vi "UpdateNativePropertyMethod.vi"(1 "VI":refnum<vi>, 2 "TypeDefControl":path=path "C:/classes/ObjectAttributes.ctl", 3 "Property":string, 5 "error IO":errorcluster, 6 "GetMethod":bool) -> (19 "error out":errorcluster)   [LabVIEW 2012, in "ClassWriterNative.lvclass"]
uses:
  <resource>/Framework/Providers/Open_GDS/ClassProviders/Provider_LvNativeClass/ClassWriterNative_class/ClassWriterNative.lvclass
  <vilib>/Utility/miscctls.llb/LVPositionTypeDef.ctl
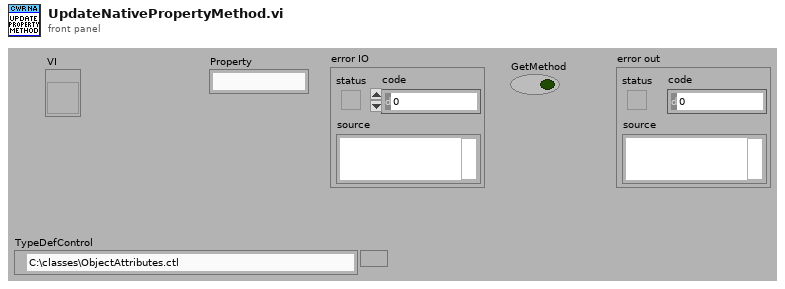
[diagram p1: front panel]
types:
  T1 = typedef "LVPositionTypeDef.ctl" = cluster{"Left":i32, "Top":i32}
  T2 = enum16{"Invalid Wire Rule", "Required", "Recommended", "Optional", "Dynamic Dispatch"}
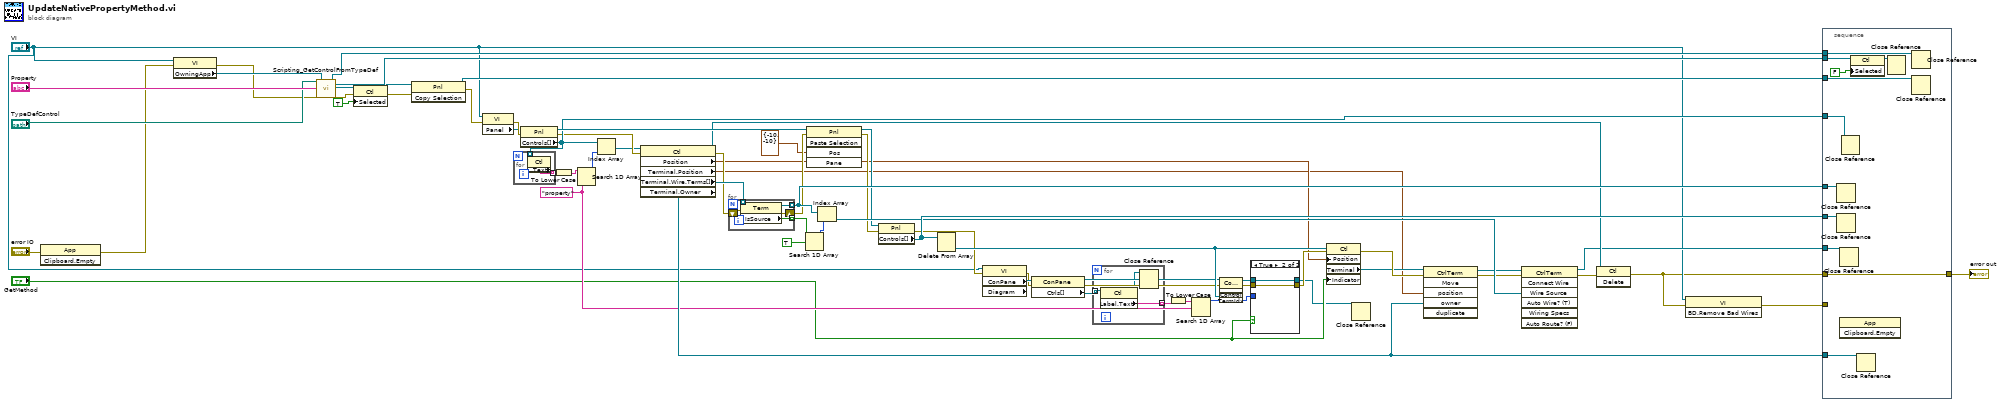
[diagram p0: block diagram]
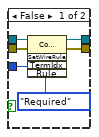
[diagram p2: hidden frame]
diagram:
  w16 = "property" ("element")
  n1 = invoke class="App" method="Clipboard.Empty"(error in="error IO") -> (error out=w5:errorcluster)  [unwired: 2 in, 2 out]
  n2 = property class="VI"(reference="VI", error in=w5) -> (error out=w4:errorcluster, "OwningApp"=w6:refnum<vi>)  [unwired: 1 out]
  n3 = call <resource>:"Scripting_GetControlFromTypeDef.vi"("TypeDefControl"="TypeDefControl", "String"="Property", "error in"=w4, "AppRef"=w6) -> ("vi reference"=w21:refnum<vi>, "Panel"=w20:refnum<vi>, "ControlRef"=w40:refnum<vi>, "error out"=w42:errorcluster)  [unwired: 12 in]
  n4 = property class="Ctl"(reference=w40, error in=w42, "Selected"=TRUE) -> (reference out=w58:refnum<vi>, error out=w41:errorcluster)
  n5 = invoke class="Pnl" method="Copy Selection"(reference=w20, error in=w41) -> (reference out=w57:refnum<vi>, error out=w43:errorcluster)  [unwired: 1 in, 1 out]
  n6 = property class="VI"(reference="VI", error in=w43) -> (error out=w45:errorcluster, "Panel"=w44:refnum<vi>)  [unwired: 1 out]
  n7 = property class="Pnl"(reference=w44, error in=w45) -> (reference out=w63:refnum<vi>, error out=w49:errorcluster, "Controls[]"=w59:refnum<vi>[])
  n8 = for {
    tunnel: w59 -> [w68] mode=indexing
    tunnel: [w67] -> w46 mode=indexing
    n9 = property class="Ctl"(reference=w68) -> ("Label.Text"=w67:string)  [unwired: 1 in, 2 out]
  }
  n10 = To Lower Case(string=w46) -> (all lower case string=w62:string[])
  n11 = Search 1D Array(1D array=w62, element=w16) -> (index of element=w47:i32)  [unwired: 1 in]
  n12 = Index Array(array=w59, index=w47) -> (element=w48:refnum<vi>)
  n13 = property class="Ctl"(reference=w48, error in=w49) -> (reference out=w34:refnum<vi>, error out=w37:errorcluster, "Position"=w29:T1, "Terminal.Position"=w24:T1, "Terminal.Wire.Terms[]"=w50:refnum<vi>[], "Terminal.Owner"=w22:refnum<vi>)
  n14 = for {
    tunnel: w50 -> [w73] mode=indexing
    tunnel: [w72] -> w51 mode=indexing
    tunnel: [w71] -> w60 mode=indexing
    shift-right: [w69] -> w36
    shift-left: w37 -> [w70]
    n15 = property class="Term"(reference=w73, error in=w70) -> (reference out=w71:refnum<vi>, error out=w69:errorcluster, "IsSource"=w72:bool)
  }
  n16 = Search 1D Array(1D array=w51, element=TRUE) -> (index of element=w53:i32)  [unwired: 1 in]
  n17 = invoke class="Pnl" method="Paste Selection"(reference=w63, error in=w36, "Pos"=T1 {"Left"=-10, "Top"=-10} ("Position")) -> (reference out=w54:refnum<vi>, error out=w33:errorcluster)  [unwired: 2 in, 3 out]
  n18 = Index Array(array=w60, index=w53) -> (element=w55:refnum<vi>)
  n19 = property class="Pnl"(reference=w54, error in=w33) -> (error out=w32:errorcluster, "Controls[]"=w61:refnum<vi>[])  [unwired: 1 out]
  n20 = Delete From Array(array=w61) -> (deleted portion=w64:refnum<vi>)  [unwired: 2 in, 1 out]
  n21 = property class="VI" props=["ConPane", "Diagram"](reference="VI", error in=w32) -> (error out=w9:errorcluster, "ConPane"=w18:refnum<vi>)  [unwired: 2 out]
  n22 = property class="ConPane"(reference=w18, error in=w9) -> (reference out=w13:refnum<vi>, error out=w12:errorcluster, "Ctrls[]"=w17:refnum<vi>[])
  n23 = for {
    tunnel: w17 -> [w75] mode=indexing
    tunnel: [w76] -> w15 mode=indexing
    n24 = property class="Ctl"(reference=w75) -> (reference out=w74:refnum<vi>, "Label.Text"=w76:string)  [unwired: 1 in, 1 out]
    n25 = Close Reference(reference=w74) -> ()  [unwired: 1 in, 1 out]
  }
  n26 = To Lower Case(string=w15) -> (all lower case string=w14:string[])
  n27 = Search 1D Array(1D array=w14, element=w16) -> (index of element=w10:i32)  [unwired: 1 in]
  n28 = invoke class="ConPane" method="AssignCtrlToTerm"(reference=w13, error in=w12, "Control"=w64, "TermIdx"=w10) -> (reference out=w65:refnum<vi>, error out=w66:errorcluster)  [unwired: 1 in, 3 out]
  n29 = case shown="True" "GetMethod" {
    tunnel: w65 -> [w82 w83]
    tunnel: w66 -> [w81 w84]
    tunnel: [w79 w84] -> w30
    tunnel: w10 -> [w78 _]
    tunnel: [w77 w83] -> w7
    frame False {
      n30 = invoke class="ConPane" method="SetWireRule"(reference=w82, error in=w81, "TermIdx"=w78, "Rule"=T2."Required") -> (reference out=w77:refnum<vi>, error out=w79:errorcluster)  [unwired: 1 in, 3 out]
    }
    frame True {
    }
  }
  n31 = property class="Ctl"(reference=w64, error in=w30, "Position"=w29, "Indicator"="GetMethod") -> (error out=w27:errorcluster, "Terminal"=w26:refnum<vi>)  [unwired: 1 out]
  n32 = Close Reference(reference=w7) -> ()  [unwired: 1 in, 1 out]
  n33 = invoke class="CtrlTerm" method="Move"(reference=w26, error in=w27, "position"=w24, "owner"=w22) -> (reference out=w25:refnum<vi>, error out=w23:errorcluster)  [unwired: 2 in, 4 out]
  n34 = invoke class="CtrlTerm" method="Connect Wire"(reference=w25, error in=w23, "Wire Source"=w55) -> (reference out=w28:refnum<vi>, error out=w35:errorcluster)  [unwired: 4 in, 5 out]
  n35 = invoke class="Ctl" method="Delete"(reference=w34, error in=w35) -> (error out=w2:errorcluster)  [unwired: 1 in, 2 out]
  n36 = invoke class="VI" method="BD.Remove Bad Wires"(reference="VI", error in=w2) -> (error out=w1:errorcluster)  [unwired: 1 in, 2 out]
  n37 = stacked-sequence {
    tunnel: w2 -> [w95]
    tunnel: [w95] -> w56
    tunnel: w21 -> [w94]
    tunnel: w57 -> [w93]
    tunnel: w58 -> [w89]
    tunnel: w59 -> [w87]
    tunnel: w60 -> [w86]
    tunnel: w61 -> [w85]
    tunnel: w28 -> [w92]
    tunnel: w22 -> [w91]
    tunnel: w1 -> [_]
    frame #0 {
      n38 = Close Reference(reference=w86) -> ()  [unwired: 1 in, 1 out]
      n39 = Close Reference(reference=w85) -> ()  [unwired: 1 in, 1 out]
      n40 = Close Reference(reference=w92) -> ()  [unwired: 1 in, 1 out]
      n41 = invoke class="App" method="Clipboard.Empty"() -> ()  [unwired: 3 in, 3 out]
      n42 = Close Reference(reference=w87) -> ()  [unwired: 1 in, 1 out]
      n43 = property class="Ctl"(reference=w89, "Selected"=FALSE) -> (reference out=w88:refnum<vi>)  [unwired: 1 in, 1 out]
      n44 = Close Reference(reference=w91) -> ()  [unwired: 1 in, 1 out]
      n45 = Close Reference(reference=w88) -> ()  [unwired: 1 in, 1 out]
      n46 = Close Reference(reference=w94) -> ()  [unwired: 1 in, 1 out]
      n47 = Close Reference(reference=w93) -> ()  [unwired: 1 in, 1 out]
    }
  }
  "error out" <- w56
